vi "P configure.vi"() -> (1 "Multiplier 1":dbl, 2 "Offset 1":dbl, 3 "Multiplier 2":dbl, 4 "Offset 2":dbl, 6 "Multiplier 3":dbl, 7 "Offset 6":dbl, 8 "Offset 3":dbl, 9 "Offset 7":dbl, 10 "Multiplier 4":dbl, 11 "Multiplier 7":dbl, 12 "Multiplier 6":dbl, 13 "Offset 5":dbl, 14 "Multiplier 5":dbl, 15 "Offset 4":dbl)   [LabVIEW 2015]
panel:
  in  "Offset 7":dbl
  in  "Multiplier 7":dbl
  in  "OK Button":bool
  in  "Offset 6":dbl
  in  "Offset 5":dbl
  in  "Offset 4":dbl
  in  "Offset 3":dbl
  in  "Offset 2":dbl
  in  "Offset 1":dbl
  in  "Multiplier 6":dbl
  in  "Multiplier 5":dbl
  in  "Multiplier 4":dbl
  in  "Multiplier 3":dbl
  in  "Multiplier 2":dbl
  in  "Multiplier 1":dbl
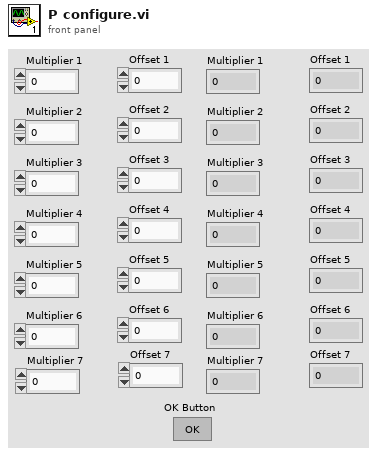
[diagram p1: front panel]
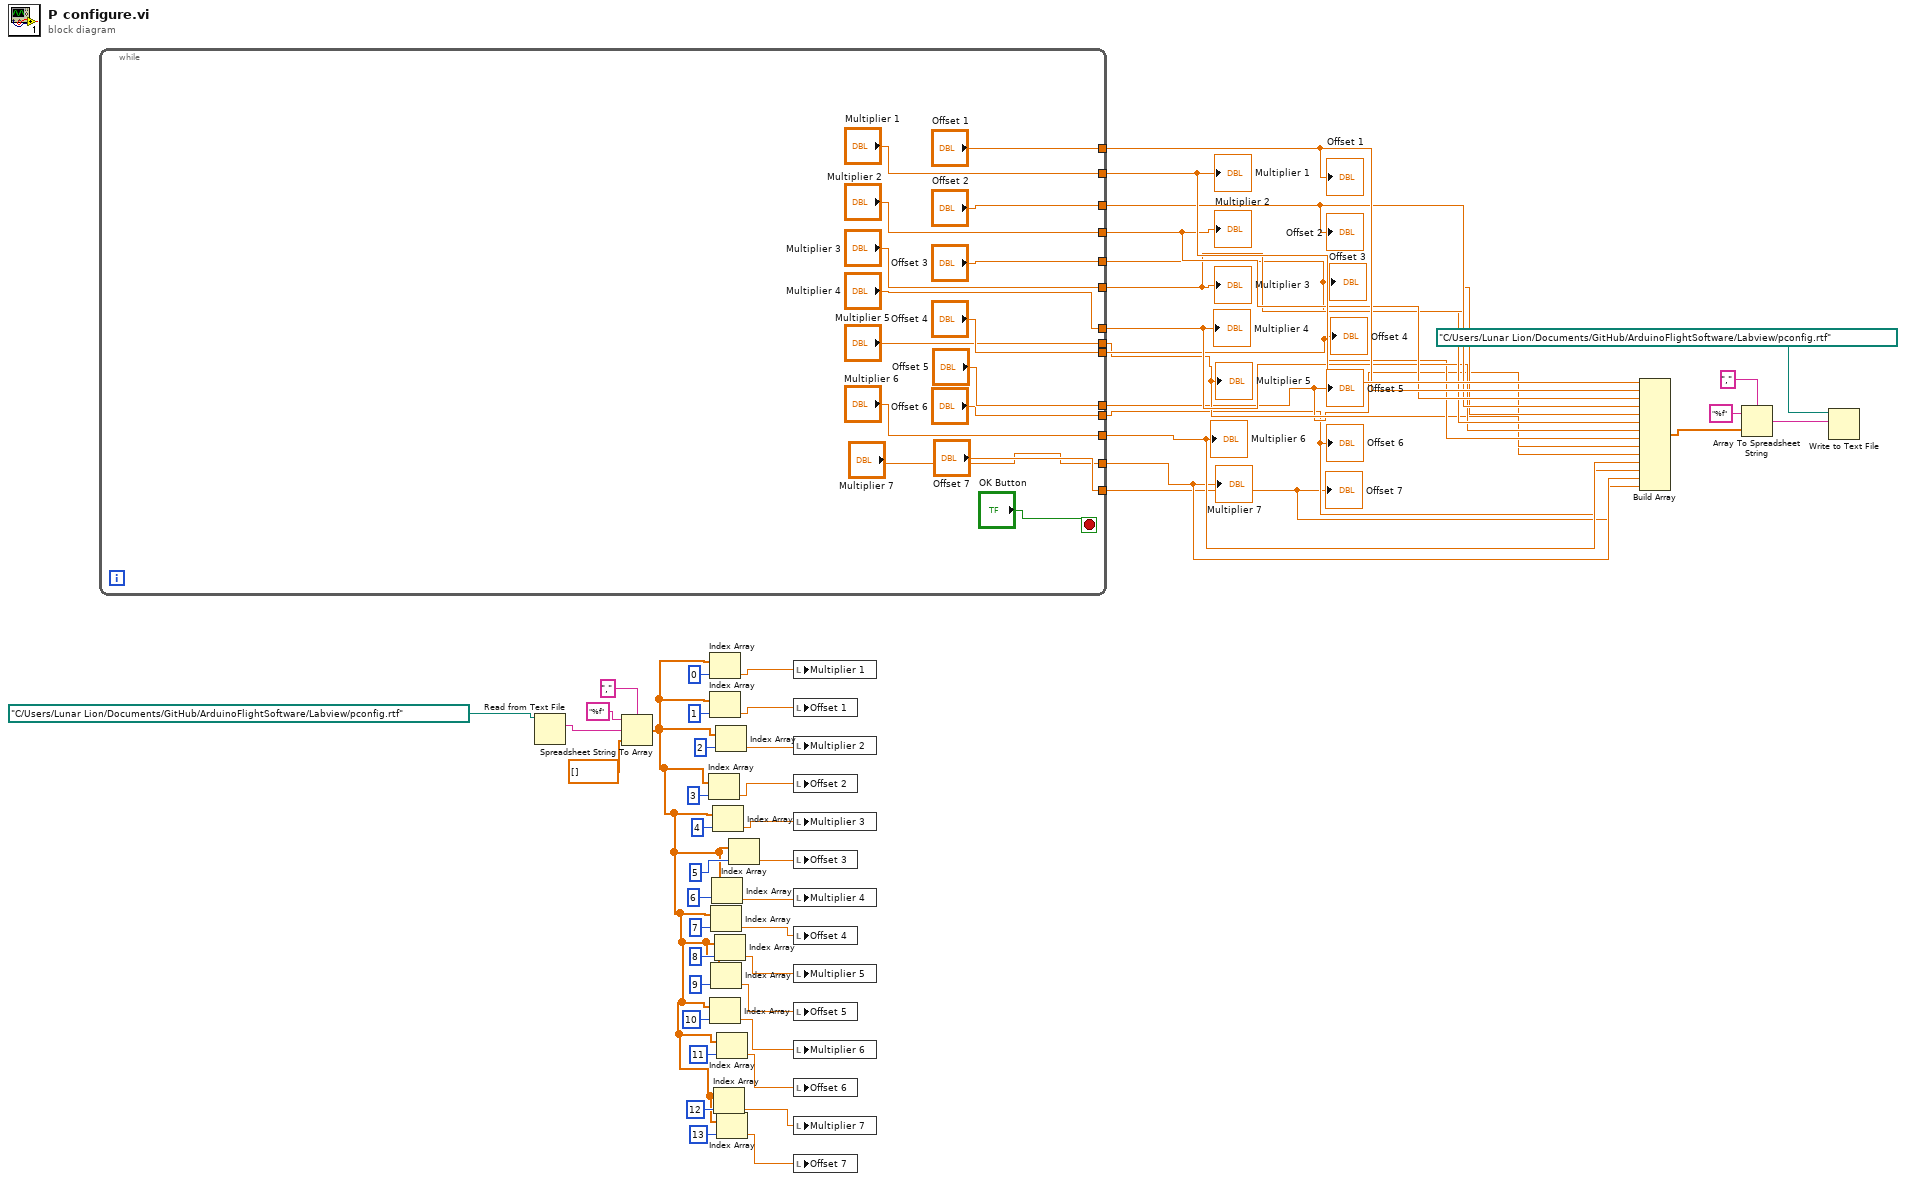
[diagram p0: block diagram]
diagram:
  n1 = while {
    tunnel: ["Multiplier 1"] -> w53
    tunnel: ["Offset 1"] -> w52
    tunnel: ["Multiplier 2"] -> w51
    tunnel: ["Offset 2"] -> w50
    tunnel: ["Multiplier 3"] -> w49
    tunnel: ["Offset 3"] -> w48
    tunnel: ["Multiplier 4"] -> w47
    tunnel: ["Offset 4"] -> w46
    tunnel: ["Multiplier 5"] -> w45
    tunnel: ["Offset 5"] -> w44
    tunnel: ["Multiplier 6"] -> w43
    tunnel: ["Offset 6"] -> w42
    tunnel: ["Offset 7"] -> w40
    tunnel: ["Multiplier 7"] -> w41
    stop <- "OK Button" stop-if-true
  }
  "Multiplier 1" <- w53
  "Multiplier 2" <- w51
  "Multiplier 3" <- w49
  "Multiplier 4" <- w47
  "Multiplier 5" <- w45
  "Multiplier 6" <- w43
  "Offset 1" <- w52
  "Offset 2" <- w50
  "Offset 3" <- w48
  "Offset 4" <- w46
  "Offset 5" <- w44
  "Offset 6" <- w42
  "Multiplier 7" <- w41
  "Offset 7" <- w40
  n2 = Read from Text File(file (use dialog)=path "C:/Users/Lunar Lion/Documents/GitHub/ArduinoFlightSoftware/Labview/pconfig.rtf") -> (text=w33:string)  [unwired: 3 in, 3 out]
  n3 = Spreadsheet String To Array(delimiter (Tab)=",", format string="%f", spreadsheet string=w33, array type (2D Dbl)=dbl[] []) -> (array=w15:dbl[])
  n4 = Index Array(array=w15, index=3) -> (element=w11:dbl)
  n5 = Index Array(array=w15, index=0) -> (element=w14:dbl)
  n6 = Index Array(array=w15, index=1) -> (element=w13:dbl)
  n7 = Index Array(array=w15, index=10) -> (element=w4:dbl)
  n8 = Index Array(array=w15, index=7) -> (element=w7:dbl)
  n9 = Index Array(array=w15, index=9) -> (element=w5:dbl)
  n10 = Index Array(array=w15, index=6) -> (element=w8:dbl)
  n11 = Index Array(array=w15, index=4) -> (element=w10:dbl)
  n12 = Index Array(array=w15, index=12) -> (element=w2:dbl)
  n13 = Index Array(array=w15, index=8) -> (element=w6:dbl)
  n14 = Index Array(array=w15, index=2) -> (element=w12:dbl)
  n15 = Index Array(array=w15, index=11) -> (element=w3:dbl)
  n16 = Index Array(array=w15, index=13) -> (element=w1:dbl)
  n17 = Index Array(array=w15, index=5) -> (element=w9:dbl)
  n18 = local write "Multiplier 1"(w14) -> ()
  n19 = local write "Offset 1"(w13) -> ()
  n20 = local write "Multiplier 2"(w12) -> ()
  n21 = local write "Offset 2"(w11) -> ()
  n22 = local write "Multiplier 3"(w10) -> ()
  n23 = local write "Offset 3"(w9) -> ()
  n24 = local write "Multiplier 4"(w8) -> ()
  n25 = local write "Offset 4"(w7) -> ()
  n26 = local write "Multiplier 5"(w6) -> ()
  n27 = local write "Offset 5"(w5) -> ()
  n28 = local write "Multiplier 6"(w4) -> ()
  n29 = local write "Offset 6"(w3) -> ()
  n30 = local write "Multiplier 7"(w2) -> ()
  n31 = local write "Offset 7"(w1) -> ()
  n32 = Build Array(w53, w52, w51, w50, w49, w48, w47, w46, w45, w44, w43, w42, w41, w40) -> (w36:dbl[])
  n33 = Array To Spreadsheet String(delimiter (Tab)=",", array=w36, 3:"%f" ("format string")) -> (spreadsheet string=w37:string)
  n34 = Write to Text File(file (use dialog)=path "C:/Users/Lunar Lion/Documents/GitHub/ArduinoFlightSoftware/Labview/pconfig.rtf", text=w37) -> ()  [unwired: 2 in, 3 out]
